vi "vertical_bar_inside_brackets_solution.vi"(8 "error in (no error)":errorcluster, 11 "Instrument Command In":string=" :TRIGger:AND:ENABle {{ON | 1} | {OFF | 0}}") -> (0 "error out":errorcluster, 3 "Instrument Command Out":string)   [LabVIEW 2018]
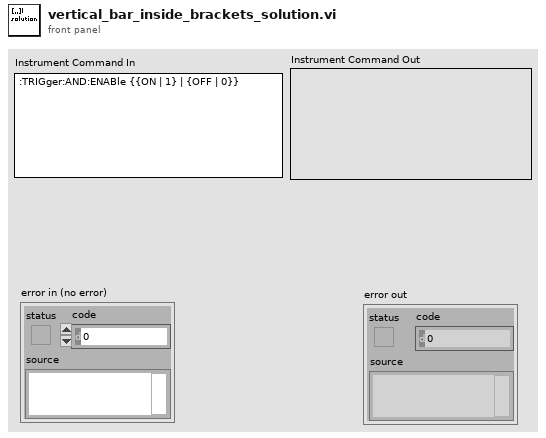
[diagram p1: front panel]
types:
  T1 = cluster{"Start Sting":string, "End String":string}[]
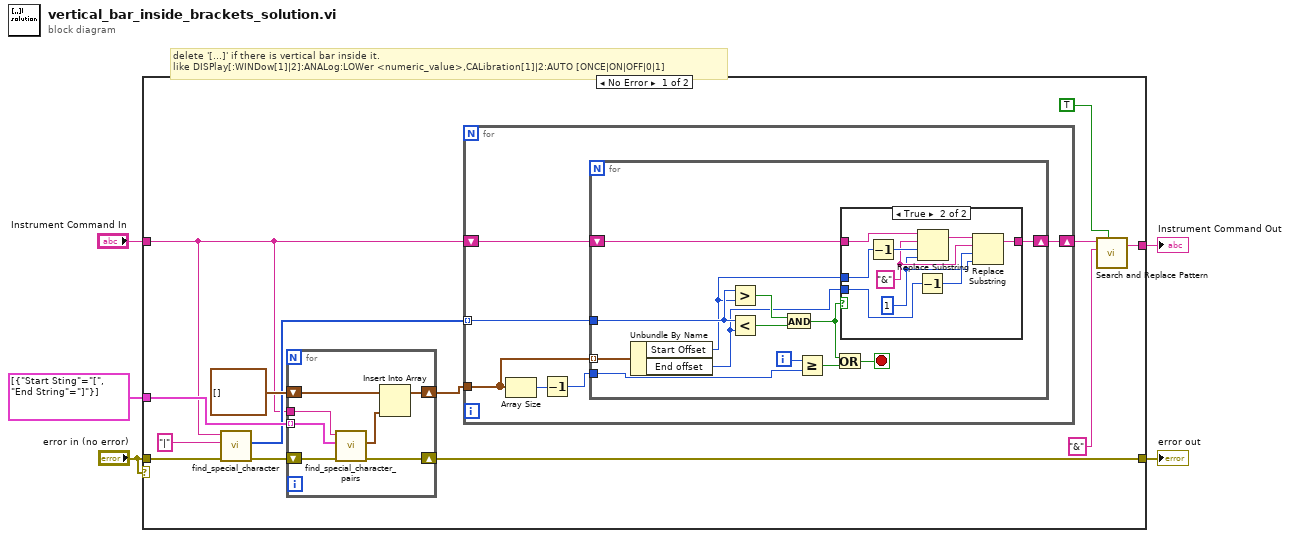
[diagram p0: block diagram]
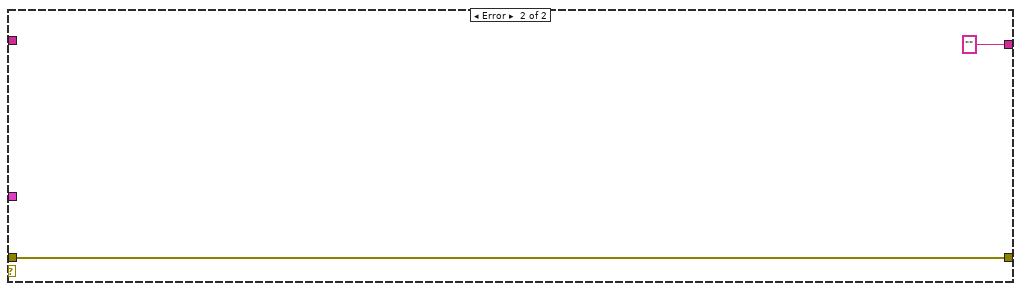
[diagram p3: hidden frame]
diagram:
  # "delete '[...]' if there is vertical bar inside it.\nlike DISPlay[:WINDow[1]|2]:ANALog:LOWer <numeric_value>,CALibration[1]|2:AUTO [ONCE|ON|OFF|0|1]"
  n1 = case shown="No Error" "error in (no error)" {
    tunnel: T1 [{"Start Sting"="[", "End String"="]"}] -> [w17 _]
    tunnel: "Instrument Command In" -> [w7 _]
    tunnel: [w9 "" ("result string")] -> w3
    tunnel: "error in (no error)" -> [w8 w56]
    tunnel: [w10 w56] -> w2
    frame No Error {
      n2 = call "find_special_character.vi"("error in (no error)"=w8, "Character"="|" ("Start Character"), "Command String"=w7) -> ("error out"=w11:errorcluster, "Offset Array"=w15:i32[])  [unwired: 7 out]
      n3 = for {
        tunnel: w7 -> [w54]
        tunnel: w17 -> [w53] mode=indexing
        shift-right: [w50] -> w14
        shift-left: cluster{"Start Offset":i32, "End offset":i32}[] [] ("Pair Offset") -> [w51]
        shift-right: [w48] -> w10
        shift-left: w11 -> [w49]
        n4 = call "find_special_character_pairs.vi"("error in (no error)"=w49, "String Pair"=w53, "Command String"=w54) -> ("error out"=w48:errorcluster, "Pair Offset"=w52:cluster{"Start Offset":i32, "End offset":i32}[])  [unwired: 7 out]
        n5 = Insert Into Array(array=w51, new element=w52) -> (w50:cluster{"Start Offset":i32, "End offset":i32}[])  [unwired: 1 in]
      }
      n6 = for {
        tunnel: w15 -> [w24] mode=indexing
        tunnel: w14 -> [w23]
        shift-right: [w19] -> w6
        shift-left: w7 -> [w20]
        n7 = Array Size(array=w23) -> (size(s)=w22:i32)
        n8 = Decrement(x=w22) -> (x-1=w21:i32)
        n9 = for {
          tunnel: w24 -> [w34]
          tunnel: w23 -> [w37] mode=indexing
          tunnel: w21 -> [w32]
          shift-right: [w25] -> w19
          shift-left: w20 -> [w28]
          i -> [w33]
          stop <- w29 stop-if-true
          n10 = Unbundle By Name(w37) -> ("Start Offset"=w27:i32, "End offset"=w26:i32)
          n11 = Greater?(x=w34, y=w27) -> (0:w36:bool)
          n12 = Less?(x=w34, y=w26) -> (x < y?=w35:bool)
          n13 = And(x=w36, y=w35) -> (x .and. y?=w31:bool)
          n14 = Greater Or Equal?(x=w33, y=w32) -> (x >= y?=w30:bool)
          n15 = Or(x=w31, y=w30) -> (x .or. y?=w29:bool)
          n16 = case shown="True" w31 {
            tunnel: w28 -> [w38 w47]
            tunnel: w27 -> [_ w46]
            tunnel: w26 -> [_ w42]
            tunnel: [w38 w40] -> w25
            frame False {
            }
            frame True {
              w43 = "&" ("substring (\"\")")
              w39 = 1 ("length (len. of substring)")
              n17 = Decrement(x=w46) -> (x-1=w45:i32)
              n18 = Decrement(x=w42) -> (x-1=w41:i32)
              n19 = Replace Substring(2:w39, 3:w45, 4:w43, 5:w47) -> (1:w44:string)  [unwired: 1 out]
              n20 = Replace Substring(2:w39, 3:w41, 4:w43, 5:w44) -> (1:w40:string)  [unwired: 1 out]
            }
          }
        }
      }
      n21 = call <vilib>:"Search and Replace Pattern.vi"("string"=w6, "regular expression (\"\")"="&" ("regular expression (\"\")"), "replace all? (F)"=TRUE) -> ("result string"=w9:string)  [unwired: 1 in, 2 out]
    }
    frame Error {
    }
  }
  "Instrument Command Out" <- w3
  "error out" <- w2
